vi "Test - Class to Cluster.vi"(8 "error in":errorcluster) -> (0 "error out":errorcluster)   [LabVIEW 2020, in "TEST - JKI JSON Object Serialization.lvlib"]
uses:
  TEST - JKI JSON Object Serialization.lvlib
  <vilib>/addons/_JKI Toolkits/Caraya/classes/Test/Test.lvclass
  source/examples/Class1/Class1.lvclass
  source/library/JKI JSON Object Serialization.lvlib
panel:
  out "JSON String":string
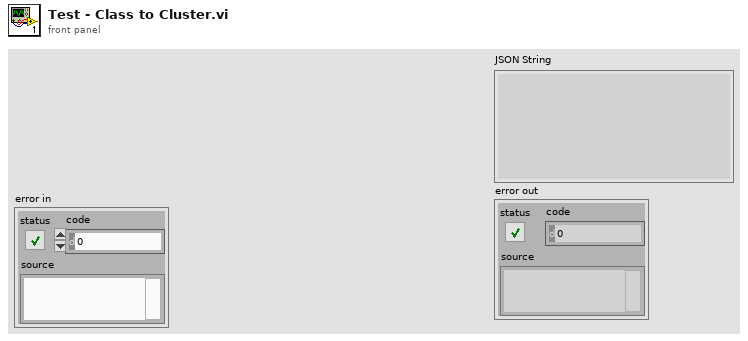
[diagram p1: front panel]
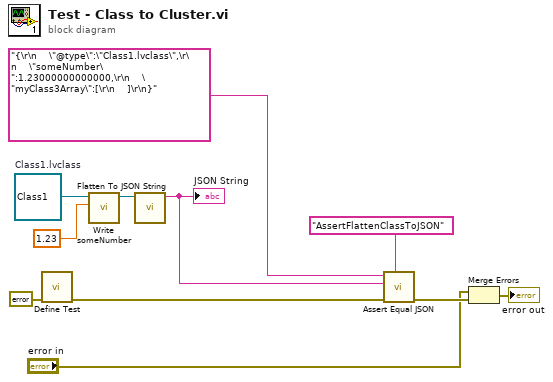
[diagram p0: block diagram]
diagram:
  w8 = refnum<class "Class1.lvclass"> refnum  # Class1.lvclass
  n1 = call <vilib>:"Define Test.vi"("error in (no error)"=errorcluster {"status"=FALSE, "code"=0, "source"=""}) -> ("error out"=w10:errorcluster)  [unwired: 9 in, 1 out]
  n2 = call-dynamic "Write someNumber.vi"("someNumber"=1.23, "Test1 in"=w8) -> ("Test1 out"=w7:refnum<class "Class1.lvclass">)  [unwired: 8 in, 1 out]
  n3 = call "Flatten To JSON String.vi"("Variant"=w7) -> ("JSON String"=w5:string)  [unwired: 9 in, 1 out]
  "JSON String" <- w5
  n4 = call "Assert Equal JSON.vi"("Label"="AssertFlattenClassToJSON" ("Label (VI Title)"), "error in (no error)"=w10, "JSON String Y"=w5, "JSON String X"="{\r\n    \"@type\":\"Class1.lvclass\",\r\n    \"someNumber\":1.23000000000000,\r\n    \"myClass3Array\":[\r\n    ]\r\n}" ("JSON String")) -> ("error out"=w11:errorcluster)  [unwired: 7 in]
  n5 = Merge Errors("error in", w11) -> (→"error out":errorcluster)
